vi "Square Waves.vi"(11 "Error In":errorcluster) -> ()   [LabVIEW 2019]
uses:
  <vilib>/Platform/TimedLoop/XDataNode/timing_clust.ctl
  <vilib>/Platform/TimedLoop/XDataNode/nitl_modes.ctl
  <vilib>/Platform/TimedLoop/XDataNode/wakeup.ctl
  Global.vi
  <vilib>/platform/TimedLoop/XDataNode/XDataNode.xnode
  <vilib>/Analysis/NI_AALBase.lvlib
  <vilib>/Platform/TimedLoop/XDataNode/XDNodeRunTimeDep.lvlib
panel:
  out "duty cycle (%) 2":dbl=50.0 format="%0.2f"
  out "frequency 2":dbl=1.0 format="%0.4e"
  out "Square wave vector":dbl[](graph)
  out "Actuator signals":cluster{dbl, dbl}(graph)
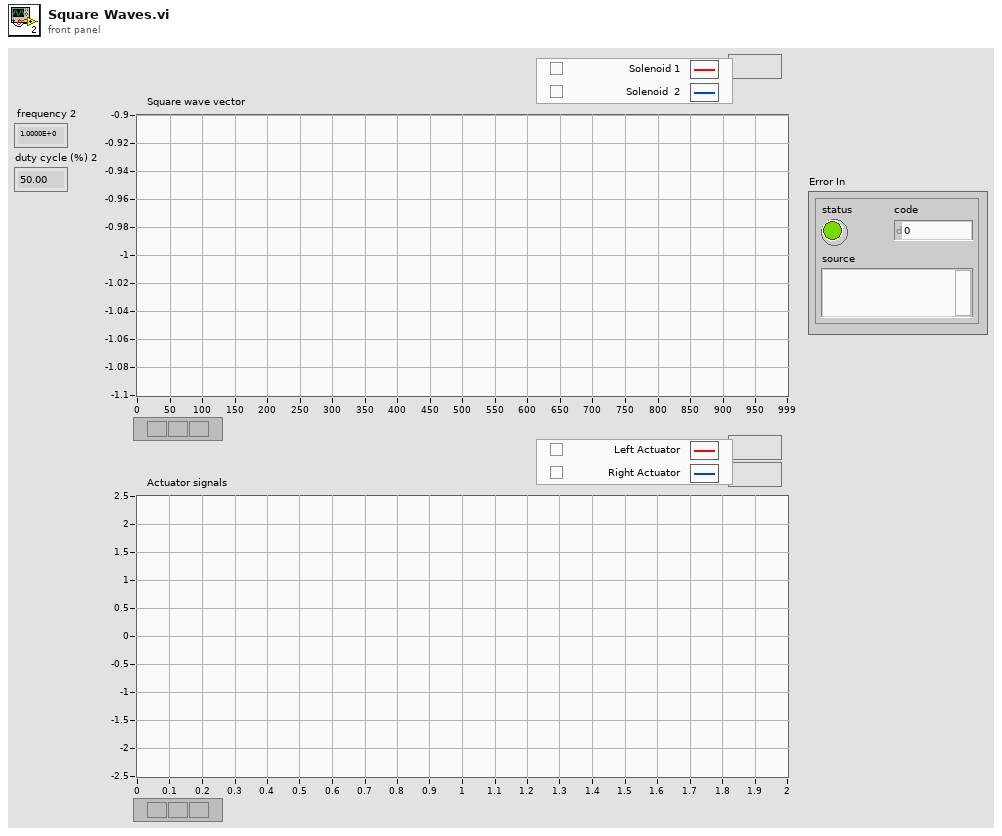
[diagram p1: front panel]
types:
  T1 = typedef "XDNodeRunTimeDep.lvlib/timing_clust.ctl" = cluster{"Expected End [f-1]":u64, "Actual End [f-1]":u64, "Finished Late? [f-1]":bool, "Expected End [i-1]":u64, "Actual End [i-1]":u64, "Finished Late? [i-1]":bool, "Expected Start [i]":u64, "Actual Start [i]":u64, "Expected Start [f]":u64, "Actual Start [f]":u64, "Source Name":string, "Structure Name":string, "Period":i64, "Deadline":i64, "Offset":i64, "Start":i64, "Priority":i32, "Timeout":i32, "Mode":T2, "Wakeup Reason":T3, "Error":errorcluster, "Source Type":string, "Secondary Source Type":string, "Global End Time":u64, "Global Start Time":u64, "Frame Duration":u64, "Iteration Duration":u64, "Assigned CPU":i32, "I/O Scan Engine Mode":u32}
  T2 = typedef "XDNodeRunTimeDep.lvlib/nitl_modes.ctl" = enum32{"No Change", "Process missed periods, maintain original phase", "Discard missed periods, maintain original phase", "Process missed periods, ignore original phase", "Discard missed periods, ignore original phase"}
  T3 = typedef "XDNodeRunTimeDep.lvlib/wakeup.ctl" = enum32{"Normal", "Aborted", "Asynchronous wakeup", "Timing source error", "Timed loop error", "Timeout"}
  T4 = cluster{"Frequency (Hz)":dbl, "Delay":dbl, "Duty cycle %":dbl}
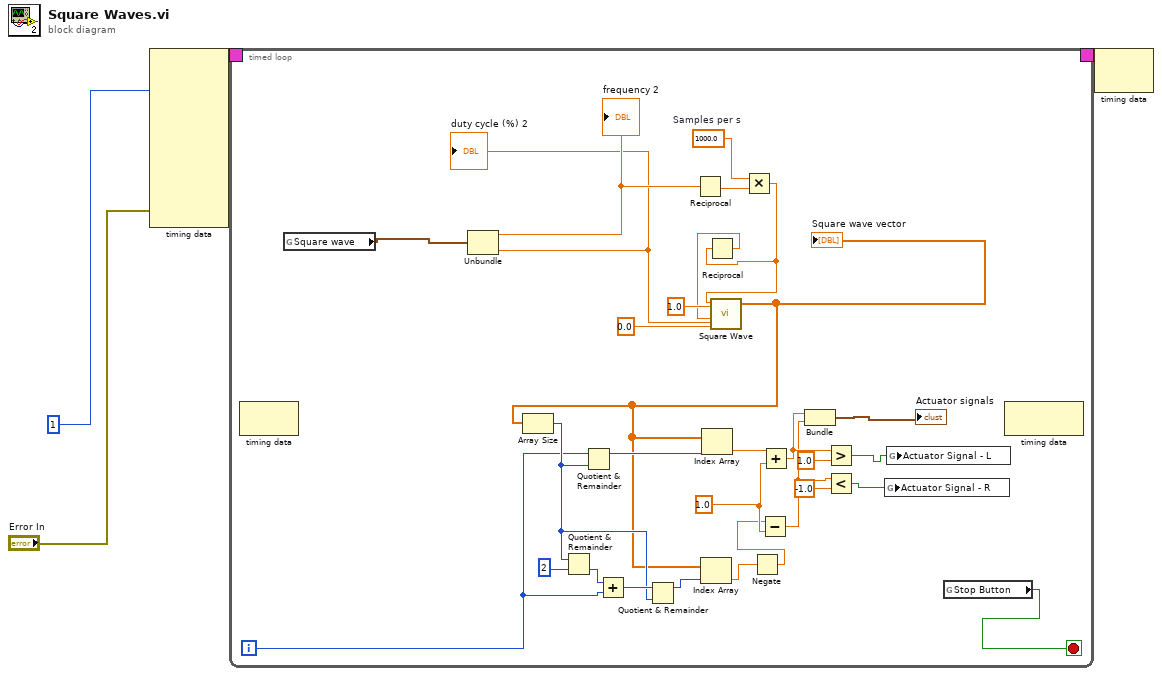
[diagram p0: block diagram]
diagram:
  n1 = node-c288(i64 1 ("Period"), "Error In") -> (w4:T1)  [unwired: 8 in]
  n2 = timed-loop {
    timing: w4 -> [_]
    timing-out: [_] -> w3
    i -> [w22]
    stop <- w15 stop-if-true
    w9 = 1000.0  # Samples per s
    w26 = 1.0 ("x")
    n3 = node-c288() -> ()  [unwired: 1 in, 1 out]
    n4 = global read "Global.vi" "Square wave"() -> (w14:T4)
    n5 = Unbundle(w14) -> ("Frequency (Hz)"=w13:dbl, "Duty cycle %"=w12:dbl)  [unwired: 1 out]
    "frequency 2" <- w13
    "duty cycle (%) 2" <- w12
    n6 = Reciprocal(x=w13) -> (1/x=w10:dbl)
    n7 = Multiply(x=w9, y=w10) -> (x*y=w8:dbl)
    n8 = Reciprocal(x=w8) -> (1/x=w7:dbl)
    n9 = call <vilib>:"Square Wave.vi"("samples"=w8, "amplitude"=1.0, "frequency"=w7, "duty cycle (%)"=w12, "phase in"=0.0) -> ("square wave"=w5:dbl[])  [unwired: 1 in, 2 out]
    "Square wave vector" <- w5
    n10 = Array Size(array=w5) -> (size(s)=w29:i32)
    n11 = Quotient & Remainder(x=w29, y=2) -> (floor(x/y)=w31:i32)  [unwired: 1 out]
    n12 = Quotient & Remainder(x=w22, y=w29) -> (x-y*floor(x/y)=w28:i32)  [unwired: 1 out]
    n13 = Add(x=w31, y=w22) -> (x+y=w30:i32)
    n14 = Quotient & Remainder(x=w30, y=w29) -> (x-y*floor(x/y)=w27:i32)  [unwired: 1 out]
    n15 = Index Array(array=w5, index=w27) -> (element=w24:dbl)
    n16 = Index Array(array=w5, index=w28) -> (element=w25:dbl)
    n17 = Negate(x=w24) -> (-x=w23:dbl)
    n18 = Subtract(x=w23, y=w26) -> (x-y=w19:dbl)
    n19 = Add(x=w25, y=w26) -> (x+y=w21:dbl)
    n20 = Bundle(w21, w19) -> (→"Actuator signals":cluster{dbl, dbl})  [unwired: 1 in]
    n21 = Greater?(x=w21, y=1.0) -> (0:w16:bool)
    n22 = Less?(x=w19, y=-1.0) -> (x < y?=w17:bool)
    n23 = global write "Global.vi" "Actuator Signal - R"(w17) -> ()
    n24 = global write "Global.vi" "Actuator Signal - L"(w16) -> ()
    n25 = global read "Global.vi" "Stop Button"() -> (w15:bool)
    n26 = node-c288() -> ()  [unwired: 1 in, 1 out]
  }
  n27 = node-c288(w3) -> ()  [unwired: 1 out]
